vi "FFT_averaging.vi"(0 "dt":dbl, 1 "freq. offset":dbl, 2 "frame":i32, 3 "current frequency":dbl, 5 "3d waveform array":dbl[][][](array[numeric]), 8 "reset frame average":bool, 10 "all frames?":bool) -> (9 "BG waveform":waveform(dbl), 11 "Mol waveform":waveform(dbl), 12 "averages compl":i32, 13 "cor waveform":waveform(dbl), 14 "BG spectrum":T1, 16 "Mol spectrum":T1, 18 "cor spectrum":T1)   [LabVIEW 2011]
doc: "Functions:\n- sums up the time domain signals\n- computes the averages over single frames or all frames\n- computes the Fourier Transform Power Spectrum \n- outputs a lot of stuff..."
uses:
  global.vi
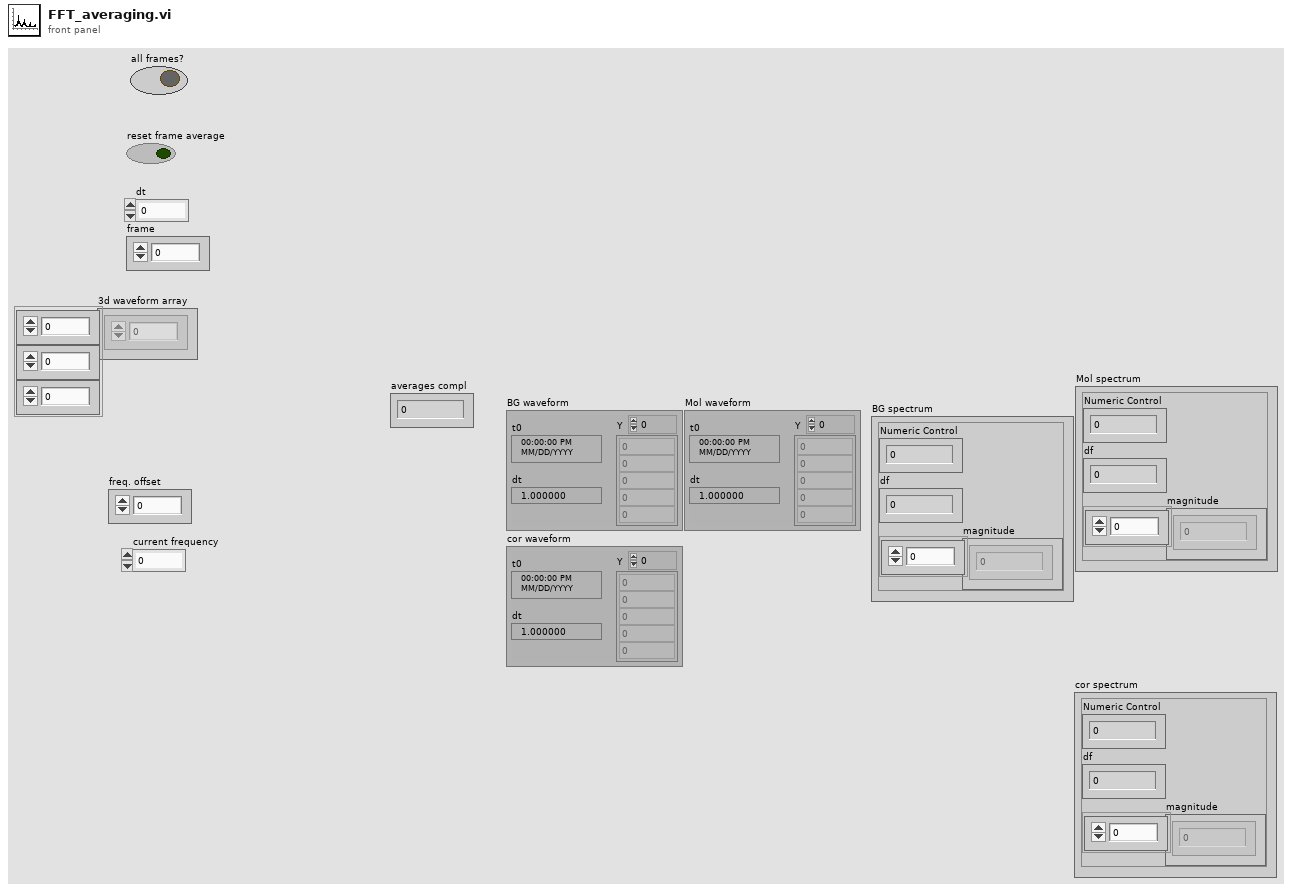
[diagram p1: front panel]
types:
  T1 = cluster{"Numeric Control":dbl, "df":dbl, "magnitude":dbl[]}
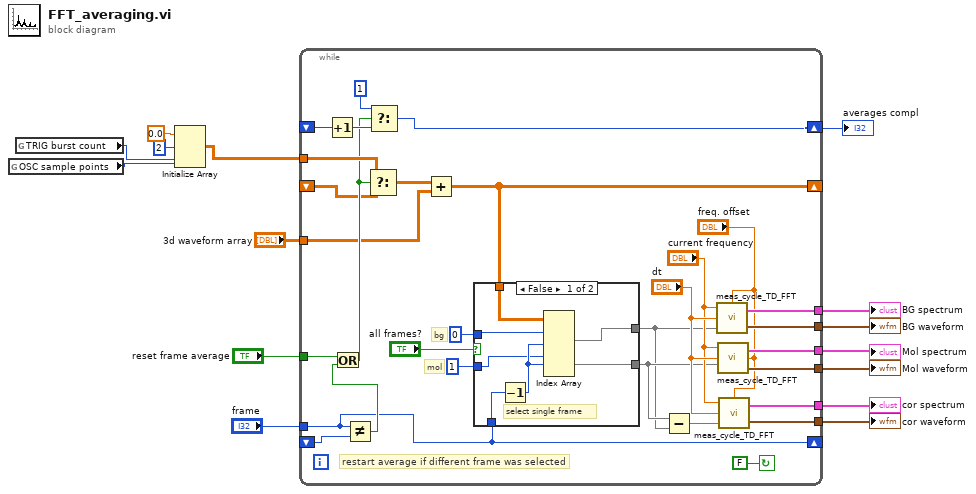
[diagram p0: block diagram]
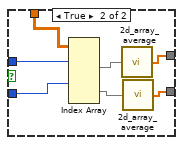
[diagram p2: hidden frame]
diagram:
  n1 = global read "global.vi" "OSC sample points"() -> (w10:i32)
  n2 = global read "global.vi" "TRIG burst count"() -> (w14:i32)
  n3 = Initialize Array(0.0 ("element"), 2 ("dimension size"), w14, w10) -> (w12:dbl[][][])
  n4 = while {
    shift-right: [w23] -> _
    shift-left: _ -> [w19]
    tunnel: w12 -> [w44]
    tunnel: "reset frame average" -> [w26]
    tunnel: "3d waveform array" -> [w20]
    shift-right: [w39] -> w9
    shift-left: _ -> [w43]
    tunnel: [w40] -> w8
    tunnel: [w41] -> w2
    tunnel: [w32] -> w1
    tunnel: [w31] -> w6
    tunnel: [w30] -> w5
    tunnel: [w29] -> w4
    tunnel: "frame" -> [w22]
    shift-right: [w22] -> _
    shift-left: _ -> [w27]
    stop <- FALSE continue-if-true
    # "restart average if different frame was selected"
    # "mol"
    # "bg"
    n5 = Increment(x=w43) -> (x+1=w42:i32)
    n6 = Not Equal?(x=w22, y=w27) -> (x != y?=w24:bool)
    n7 = Or(x=w26, y=w24) -> (x .or. y?=w25:bool)
    n8 = Select(t=w44, s=w25, f=w19) -> (s? t:f=w21:dbl[][][])
    n9 = Select(t=1, s=w25, f=w42) -> (s? t:f=w39:i32)
    n10 = Add(x=w21, y=w20) -> (x+y=w23:dbl[][][])
    n11 = case shown="False" "all frames?" {
      tunnel: [w51 w57] -> w35
      tunnel: w22 -> [w50 _]
      tunnel: [w49 w59] -> w34
      tunnel: w23 -> [w48 w55]
      tunnel: 1 ("disabled index (page)") -> [w46 w54]
      tunnel: 0 ("disabled index (page)") -> [w47 w53]
      frame False {
        # "select single frame"
        n12 = Decrement(x=w50) -> (x-1=w52:i32)
        n13 = Index Array(array=w48, index (dim 0) #1=w47, index (dim 1) #1=w52, index (dim 0) #2=w46, index (dim 1) #2=w52) -> (element #1=w49:dbl[], element #2=w51:dbl[])  [unwired: 2 in]
      }
      frame True {
        n14 = Index Array(array=w55, index (dim 0) #1=w53, index (dim 0) #2=w54) -> (element #1=w56:dbl[][], element #2=w58:dbl[][])  [unwired: 4 in]
        n15 = call "2d_array_average.vi"("2D array"=w56) -> ("array average"=w59:dbl[])  [unwired: 4 in]
        n16 = call "2d_array_average.vi"("2D array"=w58) -> ("array average"=w57:dbl[])  [unwired: 4 in]
      }
    }
    n17 = Subtract(x=w35, y=w34) -> (x-y=w33:dbl[])
    n18 = call "meas_cycle_TD_FFT.vi"("PSG freq offset"="freq. offset", "time domain array"=w34, "dt"="dt", "current frequency"="current frequency") -> ("output time domain signal"=w31:waveform(dbl), "output spectrum"=w40:T1)
    n19 = call "meas_cycle_TD_FFT.vi"("PSG freq offset"="freq. offset", "time domain array"=w35, "dt"="dt", "current frequency"="current frequency") -> ("output time domain signal"=w30:waveform(dbl), "output spectrum"=w41:T1)
    n20 = call "meas_cycle_TD_FFT.vi"("PSG freq offset"="freq. offset", "time domain array"=w33, "dt"="dt", "current frequency"="current frequency") -> ("output time domain signal"=w29:waveform(dbl), "output spectrum"=w32:T1)
  }
  "averages compl" <- w9
  "BG spectrum" <- w8
  "BG waveform" <- w6
  "Mol waveform" <- w5
  "cor waveform" <- w4
  "Mol spectrum" <- w2
  "cor spectrum" <- w1
